vi "Reorder WPs.vi"(9 "ReOrder Sim 123":i16, 11 "WP Lats and Longs Inputs":cluster{"WP LATs":dbl[], "WP LONGS":dbl[]} {"WP LONGS" format="%#_8g"; "WP LATs" format="%#_8g"}) -> (3 "WP Lats and Longs Outputs":cluster{"WP LATs":dbl[], "WP LONGS":dbl[]} {"WP LONGS" format="%#_8g"; "WP LATs" format="%#_8g"})   [LabVIEW 2014]
panel:
  # "ReOrder WPS"
  # "Inputs:"
  # "Outputs:"
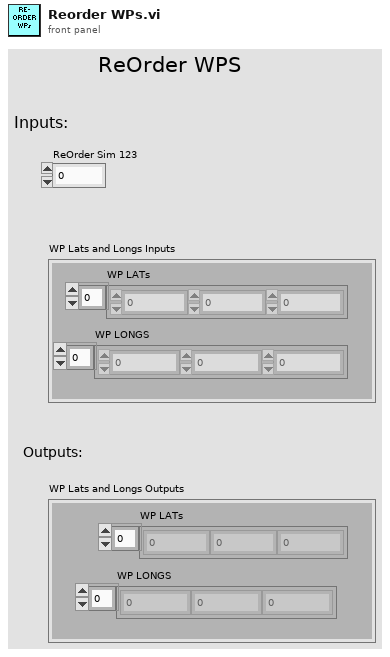
[diagram p1: front panel]
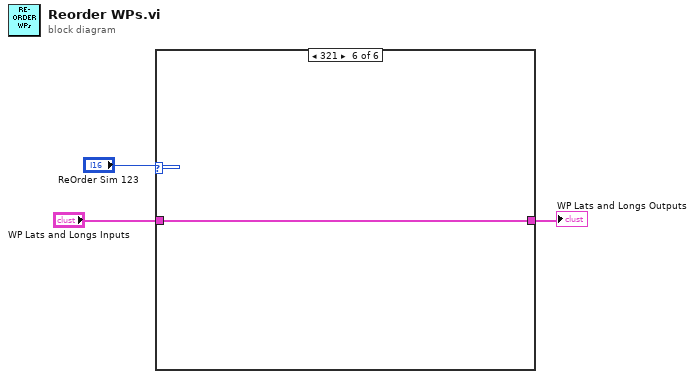
[diagram p0: block diagram]
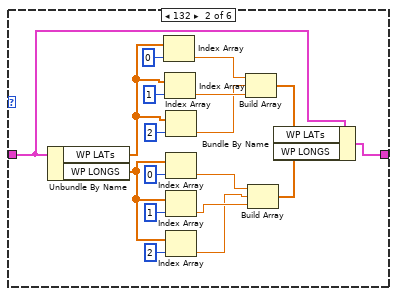
[diagram p3: hidden frame]
diagram:
  n1 = case shown="321" "ReOrder Sim 123" {
    tunnel: "WP Lats and Longs Inputs" -> [w4 w6 w23 w24 w25 w26]
    tunnel: [w4 w5 w23 w24 w25 w26] -> w1
    frame 123, Default {
    }
    frame 132 {
      n2 = Unbundle By Name(w6) -> ("WP LATs"=w19:dbl[], "WP LONGS"=w16:dbl[])
      n3 = Index Array(array=w19, index=0) -> (element=w14:dbl)
      n4 = Index Array(array=w19, index=1) -> (element=w13:dbl)
      n5 = Index Array(array=w19, index=2) -> (element=w12:dbl)
      n6 = Index Array(array=w16, index=0) -> (element=w11:dbl)
      n7 = Index Array(array=w16, index=1) -> (element=w10:dbl)
      n8 = Index Array(array=w16, index=2) -> (element=w9:dbl)
      n9 = Build Array(w14, w12, w13) -> (w8:dbl[])
      n10 = Build Array(w11, w9, w10) -> (w7:dbl[])
      n11 = Bundle By Name(cluster=w6, "WP LATs"=w8, "WP LONGS"=w7) -> (w5:cluster{"WP LATs":dbl[], "WP LONGS":dbl[]})
    }
    frame 213 {
    }
    frame 231 {
    }
    frame 312 {
    }
    frame 321 {
    }
  }
  "WP Lats and Longs Outputs" <- w1
